vi "ImaqAttributeTreeGUI.vi"(2 "error in (no error)":errorcluster, 3 "HGF_IMAQDevice":refnum<class "HGF_IMAQDevice.lvclass">) -> (0 "error out":errorcluster, 1 "dup HGF_IMAQDevice":refnum<class "HGF_IMAQDevice.lvclass">)   [LabVIEW 2014, in "HGF_VisionTools.lvlib"]
doc: "The HL Snap VI acquires an image and displays the image in an image control using the high-level acquisition VIs. A snap is appropriate for low-speed or single-capture applications where ease of programming is essential.\n\nIMAQ Init initializes the device. IMAQ Create creates an image buffer. IMAQ Snap acquires an image into the buffer, and an image control displays the image on the front panel. IMAQ Close releases resources associated with the acquisition, and the IMAQ Dispose frees the image buffer. Use this sequence to ensure that the image control displays the image before the memory is disposed."
uses:
  HGF_VisionTools.lvlib
  HGF_LVC/HGF_Auxiliary/HGF_Auxiliary.lvlib
  HGF_LVC/HGF_IMAQ/HGF_IMAQDevice/HGF_IMAQDevice.lvclass
panel:
  in  "Load":bool
  in  "Save":bool
  out "cameraName":string
  out "Units":string
  out "Tooltip":string
  in  "Attribute Tab Control":T1(tab)
  in  "U32 Value Control":u32(slide) min=576 max=16384 step=1 scale=576.0..16384.0
  in  "DBL Value Control":dbl(slide) min=0.00010395202398217064 max=1000.0 step=1.0 scale=0.00010395202398217064..1000.0
  in  "String Value Control":string
  in  "Enum Value Control":u32(ring) items=["Off", "On"]
  in  "Boolean Value Control":bool=TRUE
  in  "Command Value Control":bool
  in  "Attribute Table":string(tree)
  in  "Close":bool
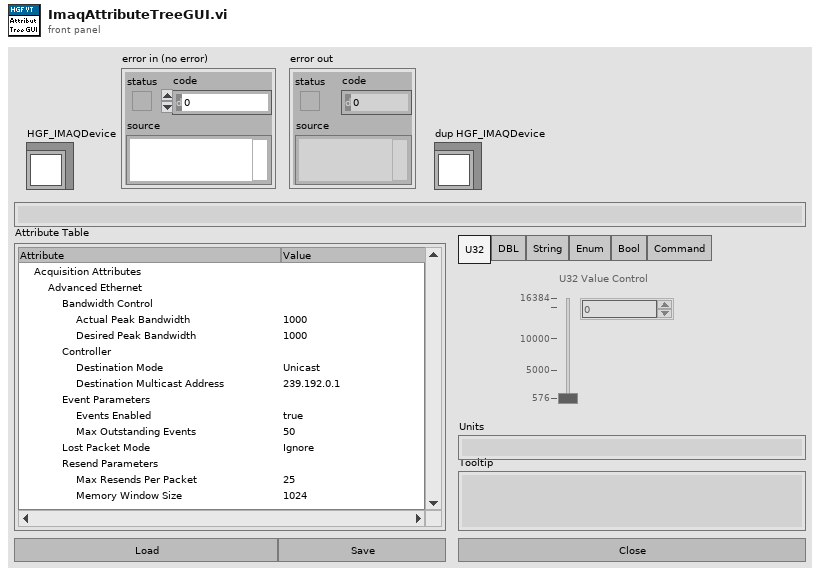
[diagram p1: front panel]
types:
  T1 = enum32{"U32", "DBL", "String", "Enum", "Bool", "Command"}
  T2 = cluster{"Attribute Tab Control":refnum<vi>, "U32 Value Control":refnum<vi>, "DBL Value Control":refnum<vi>, "String Value Control":refnum<vi>, "Enum Value Control":refnum<vi>, "Boolean Value Control":refnum<vi>, "Command Value Control":refnum<vi>}
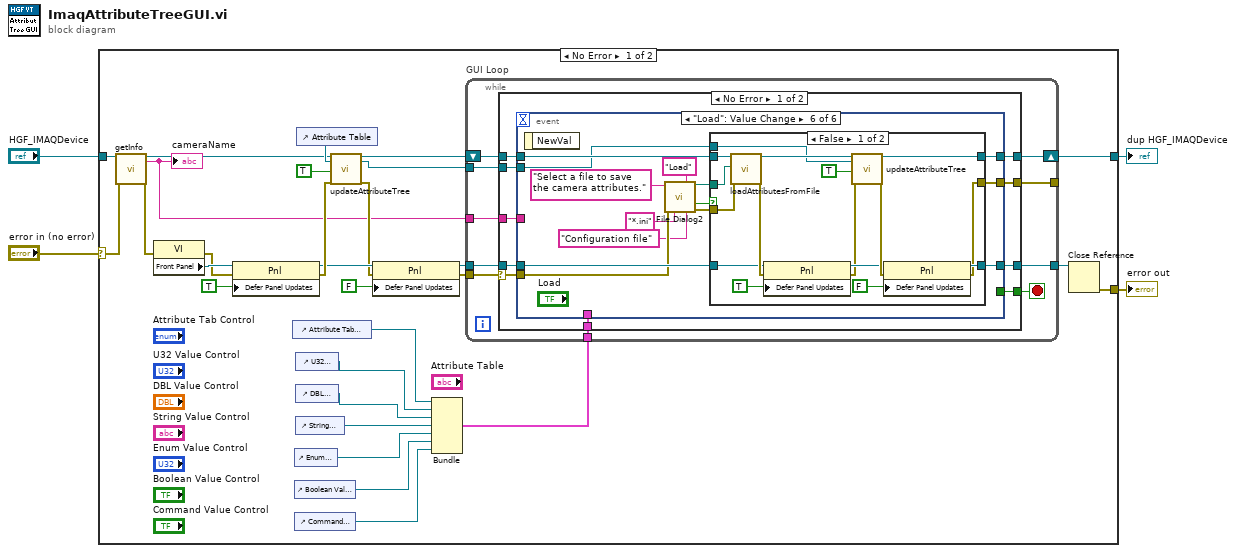
[diagram p0: block diagram]
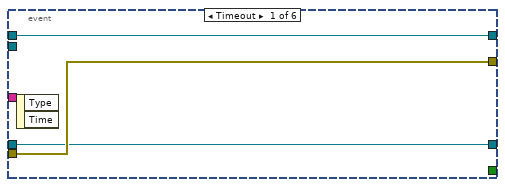
[diagram p2: hidden frame]
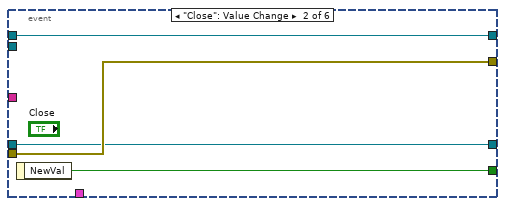
[diagram p3: hidden frame]
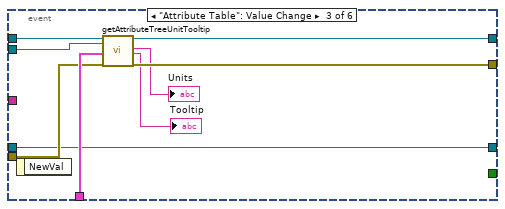
[diagram p4: hidden frame]
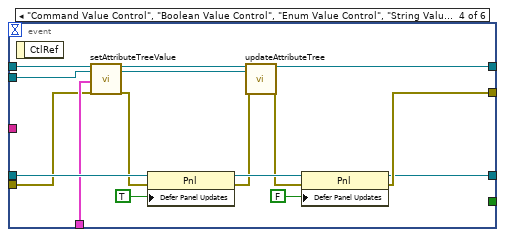
[diagram p5: hidden frame]
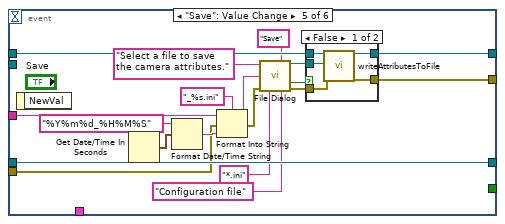
[diagram p6: hidden frame]
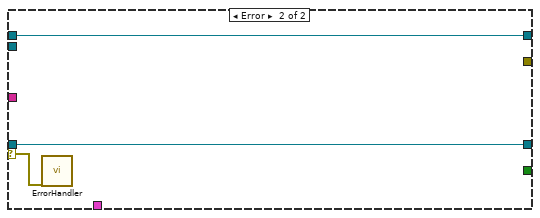
[diagram p9: hidden frame]
diagram:
  n1 = case shown="No Error" "error in (no error)" {
    selector: "error in (no error)" -> [w7 w148]
    tunnel: "HGF_IMAQDevice" -> [w9 w149]
    tunnel: [w12 w149] -> w3
    tunnel: [w10 w148] -> w1
    frame No Error {
      n2 = call "getInfo.vi"("HGF_IMAQDevice"=w9, "error in (no error)"=w7) -> ("dup HGF_IMAQDevice"=w8:refnum<class "HGF_IMAQDevice.lvclass">, "cameraName"=w5:string, "error out"=w6:errorcluster)  [unwired: 12 in, 3 out]
      "cameraName" <- w5
      n3 = property class="VI"(error in=w6) -> (error out=w11:errorcluster, "Front Panel"=w28:refnum<vi>)  [unwired: 1 in, 1 out]
      n4 = property class="Pnl"(reference=w28, error in=w11, "Defer Panel Updates"=TRUE) -> (reference out=w30:refnum<vi>, error out=w31:errorcluster)
      n5 = control-ref of="Attribute Tab Control"() -> (w17:refnum<vi>)
      n6 = control-ref of="Enum Value Control"() -> (w20:refnum<vi>)
      n7 = control-ref of="Boolean Value Control"() -> (w19:refnum<vi>)
      n8 = control-ref of="Command Value Control"() -> (w18:refnum<vi>)
      n9 = control-ref of="U32 Value Control"() -> (w23:refnum<vi>)
      n10 = control-ref of="DBL Value Control"() -> (w22:refnum<vi>)
      n11 = control-ref of="String Value Control"() -> (w21:refnum<vi>)
      n12 = control-ref of="Attribute Table"() -> (w33:refnum<vi>)
      n13 = call "updateAttributeTree.vi"("HGF_IMAQDevice"=w8, "Tree Control In"=w33, "Flush Tree?"=TRUE, "error in (no error)"=w31) -> ("dup HGF_IMAQDevice"=w25:refnum<class "HGF_IMAQDevice.lvclass">, "Tree Control Out"=w15:refnum<vi>, "error out"=w29:errorcluster)  [unwired: 13 in]
      n14 = property class="Pnl"(reference=w30, error in=w29, "Defer Panel Updates"=FALSE) -> (reference out=w14:refnum<vi>, error out=w24:errorcluster)
      n15 = Bundle("Attribute Tab Control"=w17, "U32 Value Control"=w23, "DBL Value Control"=w22, "String Value Control"=w21, "Enum Value Control"=w20, "Boolean Value Control"=w19, "Command Value Control"=w18) -> (w16:T2)  [unwired: 1 out]
      n16 = while "GUI Loop" {
        tunnel: w24 -> [w35]
        tunnel: [w41] -> _
        shift-right: [w43] -> w12
        shift-left: w25 -> [w42]
        tunnel: w16 -> [w39]
        tunnel: w15 -> [w38]
        tunnel: w14 -> [w37]
        tunnel: [w36] -> w13
        tunnel: w5 -> [w34]
        stop <- w40 stop-if-true
        n17 = case shown="No Error" w35 {
          selector: w35 -> [w45 w146]
          tunnel: [w53 w147] -> w43
          tunnel: w42 -> [w52 w147]
          tunnel: [w51 _] -> w41
          tunnel: [w50 _] -> w40
          tunnel: w39 -> [w49 _]
          tunnel: w38 -> [w48 _]
          tunnel: w37 -> [w47 w145]
          tunnel: [w46 w145] -> w36
          tunnel: w34 -> [w44 _]
          frame No Error {
            n18 = event shown="[5] \"Load\": Value Change" {
              selector: _ -> [_ _ _ _ _ _]
              dyn-events: _ -> [_ _ _ _ _ _]
              timeout: _ -> [_ _ _ _ _ _]
              tunnel: [w56 w59 w68 w75 w101 w124] -> w53
              tunnel: w52 -> [w56 w59 w69 w82 w102 w125]
              tunnel: w45 -> [w55 w58 w65 w78 w88 w114]
              tunnel: [w55 w58 w64 w71 w103 w116] -> w51
              tunnel: [_ w60 _ _ _ _] -> w50
              tunnel: w49 -> [_ _ w66 w80 _ _]
              tunnel: w48 -> [_ _ w67 w79 _ w121]
              tunnel: w47 -> [w54 w57 w61 w83 w104 w123]
              tunnel: [w54 w57 w61 w70 w104 w122] -> w46
              tunnel: w44 -> [_ _ _ _ w96 _]
              event Timeout {
                n19 = event-data() -> ()  [unwired: 1 in, 2 out]
              }
              event "Close": Value Change {
                n20 = event-data() -> ("NewVal"=w60:bool)  [unwired: 1 in]
              }
              event "Attribute Table": Value Change {
                n21 = event-data() -> ()  [unwired: 1 in, 1 out]
                n22 = call "getAttributeTreeUnitTooltip.vi"("HGF_IMAQDevice"=w69, "Tree Control In"=w67, "Tab Control Ref In"=w66, "error in (no error)"=w65) -> ("dup HGF_IMAQDevice"=w68:refnum<class "HGF_IMAQDevice.lvclass">, "Units"=→"Units":string, "Tooltip"=→"Tooltip":string, "error out"=w64:errorcluster)  [unwired: 11 in, 1 out]
              }
              event "Command Value Control", "Boolean Value Control", "Enum Value Control", "String Value Control", "DBL Value Control", "U32 Value Control": Value Change; "DBL Value Control", "U32 Value Control": Mouse Up {
                n23 = event-data() -> ()  [unwired: 1 in, 1 out]
                n24 = call "setAttributeTreeValue.vi"("HGF_IMAQDevice"=w82, "Tree Control In"=w79, "Tab Control Ref In"=w80, "error in (no error)"=w78) -> ("dup HGF_IMAQDevice"=w76:refnum<class "HGF_IMAQDevice.lvclass">, "Tree Control Out"=w72:refnum<vi>, "error out"=w77:errorcluster)  [unwired: 13 in]
                n25 = property class="Pnl"(reference=w83, error in=w77, "Defer Panel Updates"=TRUE) -> (reference out=w81:refnum<vi>, error out=w74:errorcluster)
                n26 = call "updateAttributeTree.vi"("HGF_IMAQDevice"=w76, "Tree Control In"=w72, "error in (no error)"=w74) -> ("dup HGF_IMAQDevice"=w75:refnum<class "HGF_IMAQDevice.lvclass">, "error out"=w73:errorcluster)  [unwired: 14 in, 1 out]
                n27 = property class="Pnl"(reference=w81, error in=w73, "Defer Panel Updates"=FALSE) -> (reference out=w70:refnum<vi>, error out=w71:errorcluster)
              }
              event "Save": Value Change {
                n28 = event-data() -> ()  [unwired: 1 in, 1 out]
                n29 = Get Date/Time In Seconds() -> (seconds since 1Jan1904=w89:timestamp)
                n30 = Format Date/Time String(time format string (%c)="%Y%m%d_%H%M%S", seconds (now)=w89) -> (date/time string=w92:string)  [unwired: 1 in]
                n31 = Format Into String(format string="_%s.ini", initial string=w96, error in=w88, w92) -> (resulting string=w95:string, error out=w94:errorcluster)
                n32 = call "File Dialog"("prompt"="Select a file to save the camera attributes.", "button label"="Save", "default name"=w95, "error in"=w94, "pattern (all files)"="*.ini", "pattern label"="Configuration file") -> ("selected path"=w100:path, "cancelled"=w99:bool, "error out"=w93:errorcluster)  [unwired: 6 in, 1 out]
                n33 = case shown="False" w99 {
                  tunnel: [w109 w110] -> w103
                  tunnel: w102 -> [w108 w111]
                  tunnel: [w107 w111] -> w101
                  tunnel: w100 -> [w106 _]
                  tunnel: w93 -> [w105 w110]
                  frame False {
                    n34 = call "writeAttributesToFile.vi"("HGF_IMAQDevice"=w108, "Filename"=w106, "error in (no error)"=w105) -> ("dup HGF_IMAQDevice"=w107:refnum<class "HGF_IMAQDevice.lvclass">, "error out"=w109:errorcluster)  [unwired: 15 in]
                  }
                  frame True {
                  }
                }
              }
              event "Load": Value Change {
                n35 = event-data() -> ()  [unwired: 1 in, 1 out]
                n36 = call "File Dialog2"("prompt"="Select a file to save the camera attributes.", "button label"="Load", "error in"=w114, "pattern (all files)"="*.ini", "pattern label"="Configuration file") -> ("selected path"=w117:path, "cancelled"=w118:bool, "error out"=w115:errorcluster)  [unwired: 7 in, 1 out]
                n37 = case shown="False" w118 {
                  tunnel: w125 -> [w141 w144]
                  tunnel: [w133 w144] -> w124
                  tunnel: w123 -> [w131 w142]
                  tunnel: [w130 w142] -> w122
                  tunnel: w121 -> [w129 _]
                  tunnel: w117 -> [w128 _]
                  tunnel: [w126 w143] -> w116
                  tunnel: w115 -> [w127 w143]
                  frame False {
                    n38 = call "loadAttributesFromFile.vi"("HGF_IMAQDevice"=w141, "Filename"=w128, "error in (no error)"=w127) -> ("dup HGF_IMAQDevice"=w134:refnum<class "HGF_IMAQDevice.lvclass">, "error out"=w132:errorcluster)  [unwired: 15 in]
                    n39 = property class="Pnl"(reference=w131, error in=w132, "Defer Panel Updates"=TRUE) -> (reference out=w137:refnum<vi>, error out=w136:errorcluster)
                    n40 = call "updateAttributeTree.vi"("HGF_IMAQDevice"=w134, "Tree Control In"=w129, "Flush Tree?"=TRUE, "error in (no error)"=w136) -> ("dup HGF_IMAQDevice"=w133:refnum<class "HGF_IMAQDevice.lvclass">, "error out"=w138:errorcluster)  [unwired: 13 in, 1 out]
                    n41 = property class="Pnl"(reference=w137, error in=w138, "Defer Panel Updates"=FALSE) -> (reference out=w130:refnum<vi>, error out=w126:errorcluster)
                  }
                  frame True {
                  }
                }
              }
            }
          }
          frame Error {
            n42 = call "ErrorHandler.vi"("error in (no error)"=w146) -> ()  [unwired: 6 in, 13 out]
          }
        }
      }
      n43 = Close Reference(reference=w13) -> (error out=w10:errorcluster)  [unwired: 1 in]
    }
    frame Error {
    }
  }
  "dup HGF_IMAQDevice" <- w3
  "error out" <- w1
